vi "Calibrate Adjust Sense Data Query.vi"(8 "error in (no error)":errorcluster, 11 "VISA resource name":refnum<visa-resource-name>="GPIB0::24::INSTR") -> (0 "error out":errorcluster, 2 "Sense Data":string, 3 "VISA resource name out":refnum<visa-resource-name>)   [LabVIEW 2022 SP3, in "Keithley 2450.lvlib"]
doc: "Returns calibration adjust sense data."
uses:
  Keithley 2450.lvlib
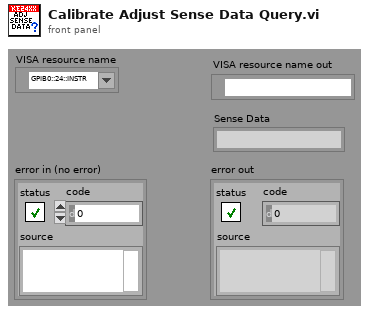
[diagram p1: front panel]
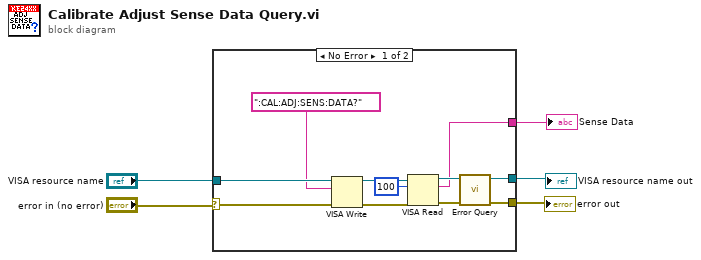
[diagram p0: block diagram]
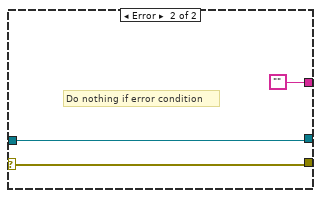
[diagram p2: hidden frame]
diagram:
  n1 = case shown="No Error" "error in (no error)" {
    selector: "error in (no error)" -> [w16 w19]
    tunnel: [w14 w19] -> w2
    tunnel: "VISA resource name" -> [w15 w18]
    tunnel: [w13 w18] -> w3
    tunnel: [w7 ""] -> w1
    frame No Error {
      n2 = VISA Write(VISA resource name=w15, write buffer=":CAL:ADJ:SENS:DATA?" ("string"), error in (no error)=w16) -> (VISA resource name out=w9:refnum<visa-resource-name>, error out=w8:errorcluster)  [unwired: 1 out]
      n3 = VISA Read(VISA resource name=w9, byte count=u32 100, error in (no error)=w8) -> (VISA resource name out=w10:refnum<visa-resource-name>, read buffer=w7:string, error out=w11:errorcluster)  [unwired: 1 out]
      n4 = call "Error Query.vi"("error in (no error)"=w11, "VISA resource name"=w10) -> ("error out"=w14:errorcluster, "VISA resource name out"=w13:refnum<visa-resource-name>)  [unwired: 6 in, 2 out]
    }
    frame Error {
      # "Do nothing if error condition"
    }
  }
  "error out" <- w2
  "VISA resource name out" <- w3
  "Sense Data" <- w1
